vi "EneryPixelInit.vi"(8 "error in (no error)":errorcluster, 11 "MagSpec_Bella in":refnum<class "MagSpec_Bella.lvclass">) -> (0 "error out":errorcluster, 3 "MagSpec_Bella out":refnum<class "MagSpec_Bella.lvclass">)   [LabVIEW 2013, in "MagSpec_Bella.lvclass"]
uses:
  MagSpec_Bella.lvclass
  MagSpec_Bella.lvclass/MagSpec_Bella.ctl
panel:
  out "Charge Compensation 2":dbl[][](graph)
  out "energy dep":dbl[][](graph)
  out "Bending angle":dbl[][](graph)
  out "Charge Compensation":dbl[][](graph)
  out "Momentum [MeV/C]":dbl[][](graph)
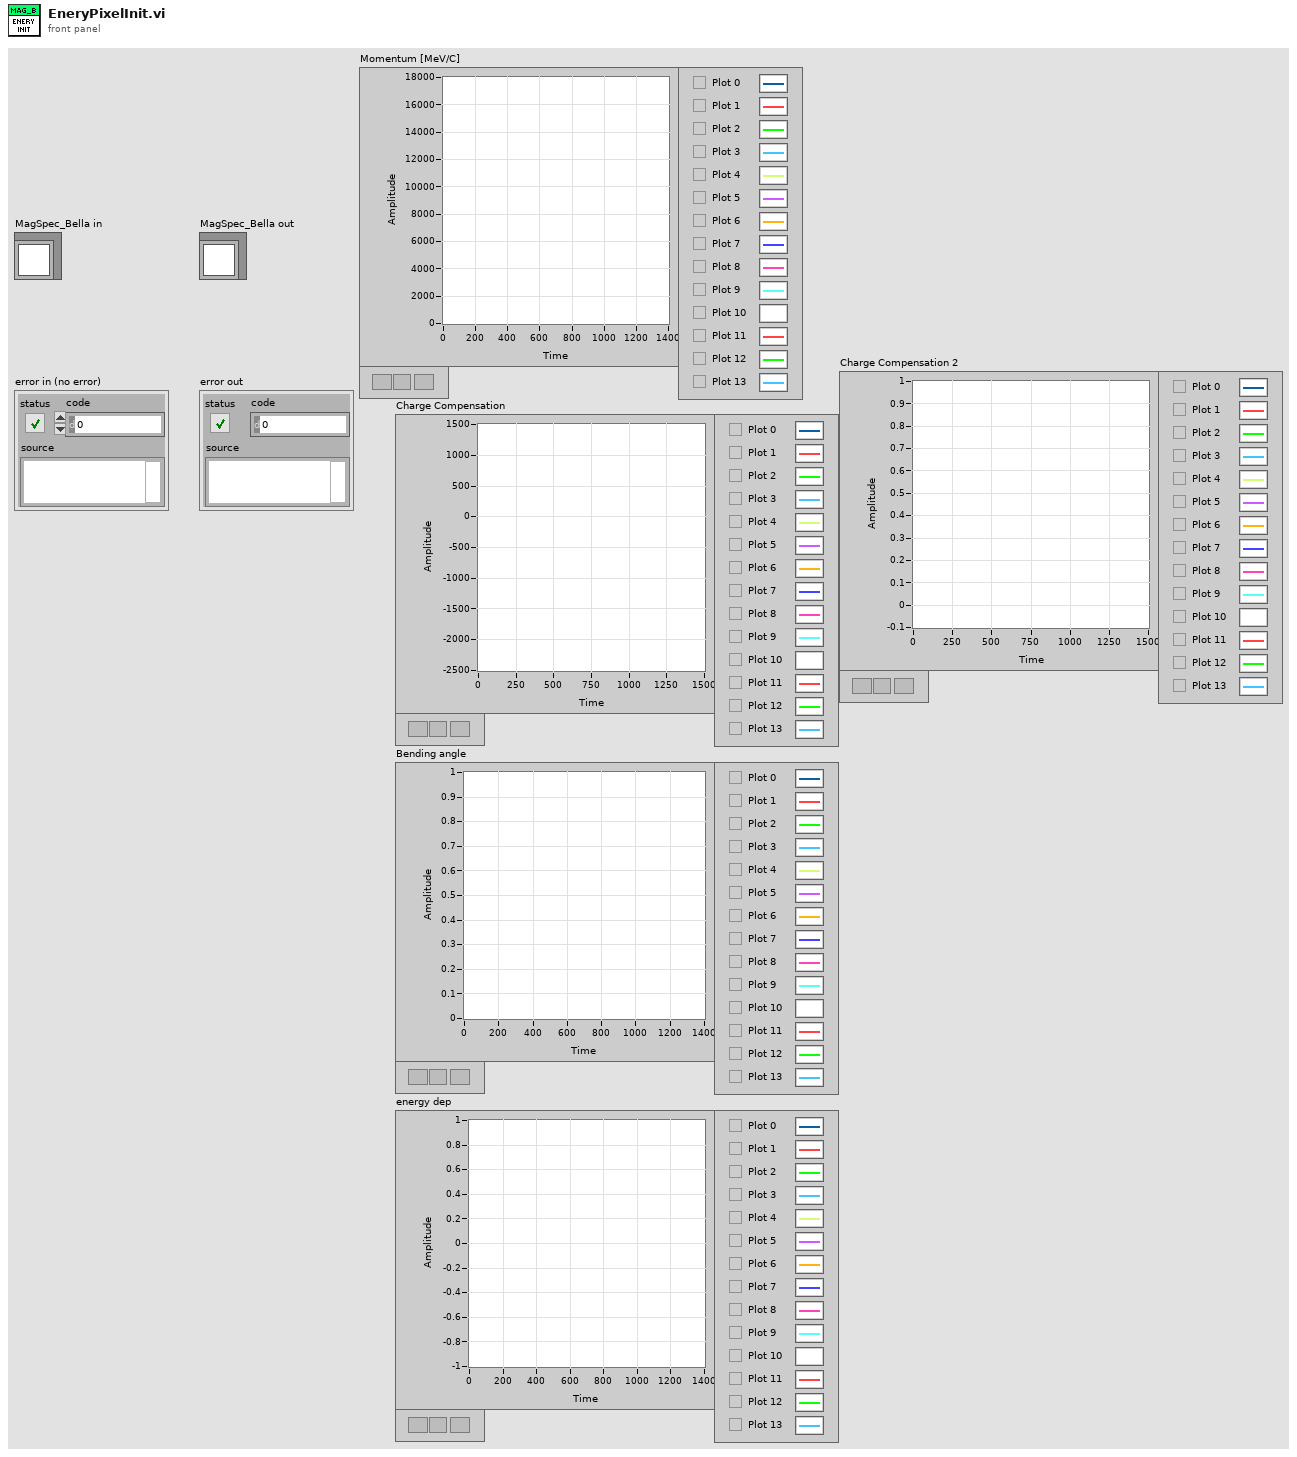
[diagram p1: front panel]
types:
  T1 = typedef "Calibration_Pixel_based.ctl" = cluster{"y1(pixel)":dbl[], "y2(pixel)":dbl[], "dp/B [MeV/C/B] (pixel)":dbl[], "energyDependence Input(pixel)":dbl[], "bending angle [deg](pixel)":dbl[], "total path(pixel)":dbl[], "pixel angle (y)(pixel)":dbl[], "energy dependence (pixel)":dbl[], "charge compensation (pixel)":dbl[], "Momentum [MeV/C](pixel)":dbl[], "angular compensation(pixel)":dbl[]}
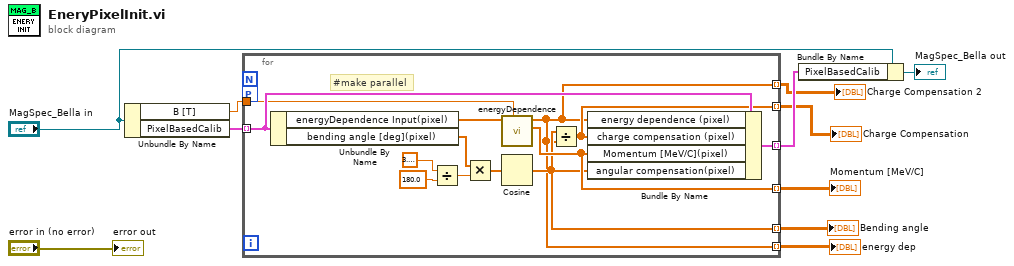
[diagram p0: block diagram]
diagram:
  n1 = Unbundle By Name("MagSpec_Bella in") -> ("B [T]"=w6:dbl, "PixelBasedCalib"=w7:T1[])
  n2 = for {
    tunnel: w7 -> [w17] mode=indexing
    tunnel: [w18] -> w8 mode=indexing
    tunnel: w6 -> [w16]
    tunnel: [w15] -> w5 mode=indexing
    workers-P: _ -> [_]
    tunnel: [w14] -> w4 mode=indexing
    tunnel: [w13] -> w3 mode=indexing
    tunnel: [w12] -> w2 mode=indexing
    tunnel: [w12] -> w1 mode=indexing
    # "#make parallel"
    n3 = Unbundle By Name(w17) -> ("energyDependence Input(pixel)"=w23:dbl[], "bending angle [deg](pixel)"=w24:dbl[])
    n4 = Divide(x=3.141592653589793, y=180.0) -> (x/y=w20:dbl)
    n5 = Multiply(x=w24, y=w20) -> (x*y=w19:dbl[])
    n6 = call "energyDependence.vi"("B [T]"=w16, "energy vs pixel"=w23) -> ("Momentum [MeV/C] vs pix"=w15:dbl[], "energy dependence"=w12:dbl[])  [unwired: 8 in]
    n7 = Cosine(x=w19) -> (cos(x)=w13:dbl[])
    n8 = Divide(x=w13, y=w12) -> (x/y=w14:dbl[])
    n9 = Bundle By Name(cluster=w17, "energy dependence (pixel)"=w12, "charge compensation (pixel)"=w14, "Momentum [MeV/C](pixel)"=w15, "angular compensation(pixel)"=w13) -> (w18:T1)
  }
  "Momentum [MeV/C]" <- w5
  "Charge Compensation" <- w4
  "Bending angle" <- w3
  "energy dep" <- w2
  "Charge Compensation 2" <- w1
  n10 = Bundle By Name(cluster="MagSpec_Bella in", "PixelBasedCalib"=w8) -> (→"MagSpec_Bella out":refnum<class "MagSpec_Bella.lvclass">)
  "error out" <- "error in (no error)"
